vi "实时小时数据单参数上传2.vi"(11 "错误输入（无错误）":errorcluster) -> (4 "数据发送起始时间":timestamp format="%<%.3X\n%Y/%m/%d>T", 15 "error out":errorcluster)   [LabVIEW 2016, in "数据传输系统-04.lvlib"]
uses:
  <vilib>/Utility/config.llb/Read Key (String).vi
  <vilib>/Utility/config.llb/Write Key (String).vi
  <vilib>/Utility/config.llb/NI_LVConfig.lvlib
panel:
  out "数据拆分":bool
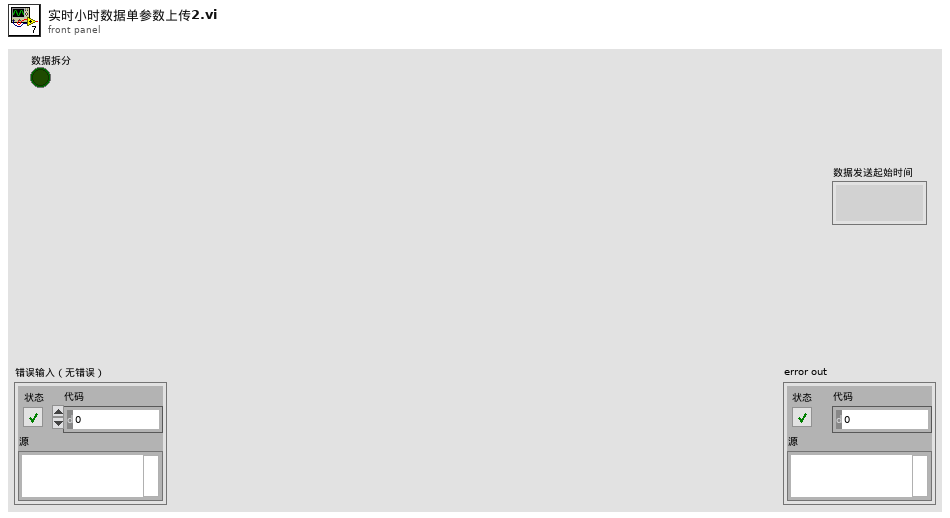
[diagram p1: front panel]
types:
  T1 = cluster{"CODMn":string, "CODCr":string, "DO":string, "铜":string, "PH":string, "氨氮":string, "比电导率":string, "水温":string, "COD":string, "浊度":string, "总氮":string, "总磷":string, "叶绿素a":string, "藻密度":string, "水位":string, "流速":string, "方向":string, "瞬时流量":string, "累积流量":string, "正累积流量":string, "负累积流量":string, "亚硝酸盐":string, "硫化物":string, "ORP":string, "铅":string, "镉":string, "锌":string, "镍":string, "锰":string, "汞":string, "气温":string, "气压":string, "风速":string, "风向":string, "空气温度":string, "相对湿度":string, "分钟雨量":string, "小时雨量":string, "日雨量":string, "累积雨量":string, "盐度":string, "磷酸盐":string, "硝氮":string, "氟化物":string, "挥发酚":string, "氯化物":string, "蓝绿藻":string, "余氯":string, "综合生物毒性":string, "艏向":string, "横摇":string, "纵摇":string, "分层标志":string, "层状态1":string, "层状态2":string, "水平平均流速":string, "流向":string, "北向流速分量":string, "东向流速分量":string, "垂直流速分量":string, "最大波高":string, "最大波周期":string, "1/10波高":string, "1/10波周期":string, "有效波高":string, "有效波周期":string, "平均波高":string, "平均波周期":string, "波向":string, "波个数":string, "水深":string, "X轴流速":string, "Y轴流速":string, "信号强度":string, "电压":string, "悬浮物":string}
  T2 = cluster{"setini":string, "sysini":string, "hechaini":string, "actualwrite":string, "actualread":string, "datasent":string, "反控命令信息队列":string, "反控与仪器交互":string}
  T3 = typedef "NI_LVConfig.lvlib/Config Data RefNum.ctl" = refnum<k1>
  T4 = cluster{"time1":string, "time2":string, "time3":string, "time4":string, "time5":string, "time6":string, "time7":string, "time8":string, "time9":string, "time10":string, "time11":string, "time12":string, "time13":string, "time14":string, "time15":string, "time16":string, "time17":string, "time18":string, "time19":string, "time20":string, "time21":string, "time22":string, "time23":string, "time24":string, "time25":string, "time26":string, "time27":string, "time28":string, "time29":string, "time30":string, "time31":string, "time32":string, "time33":string, "time34":string, "time35":string, "time36":string, "time37":string, "time38":string, "time39":string, "time40":string, "time41":string, "time42":string, "time43":string, "time44":string, "time45":string, "time46":string, "time47":string, "time48":string, "time49":string, "time50":string, "time51":string, "time52":string, "time53":string, "time54":string, "time55":string, "time56":string, "time57":string, "time58":string, "time59":string, "time60":string, "time61":string, "time62":string, "time63":string, "time64":string, "time65":string, "time66":string, "time67":string, "time68":string, "time69":string, "time70":string, "time71":string, "time72":string, "time73":string, "time74":string, "time75":string, "time76":string}
  T5 = cluster{"水样数据索引[0]":string, "水样数据索引[1]":string, "水样数据索引[2]":string, "水样数据索引[3]":string, "水样数据索引[4]":string, "水样数据索引[5]":string, "水样数据索引[6]":string, "水样数据索引[7]":string, "水样数据索引[8]":string, "水样数据索引[9]":string, "水样数据索引[10]":string, "水样数据索引[11]":string, "水样数据索引[12]":string, "水样数据索引[13]":string, "水样数据索引[14]":string, "水样数据索引[15]":string, "水样数据索引[16]":string, "水样数据索引[17]":string, "水样数据索引[18]":string, "水样数据索引[19]":string, "水样数据索引[20]":string, "水样数据索引[21]":string, "水样数据索引[22]":string, "水样数据索引[23]":string, "水样数据索引[24]":string, "水样数据索引[25]":string, "水样数据索引[26]":string, "水样数据索引[27]":string, "水样数据索引[28]":string, "水样数据索引[29]":string, "水样数据索引[30]":string, "水样数据索引[31]":string, "水样数据索引[32]":string, "水样数据索引[33]":string, "水样数据索引[34]":string, "水样数据索引[35]":string, "水样数据索引[36]":string, "水样数据索引[37]":string, "水样数据索引[38]":string, "水样数据索引[39]":string, "水样数据索引[40]":string, "水样数据索引[41]":string, "水样数据索引[42]":string, "水样数据索引[43]":string, "水样数据索引[44]":string, "水样数据索引[45]":string, "水样数据索引[46]":string, "水样数据索引[47]":string, "水样数据索引[48]":string, "水样数据索引[49]":string, "水样数据索引[50]":string, "水样数据索引[51]":string, "水样数据索引[52]":string, "水样数据索引[53]":string, "水样数据索引[54]":string, "水样数据索引[55]":string, "水样数据索引[56]":string, "水样数据索引[57]":string, "水样数据索引[58]":string, "水样数据索引[59]":string, "水样数据索引[60]":string, "水样数据索引[61]":string, "水样数据索引[62]":string, "水样数据索引[63]":string, "水样数据索引[64]":string, "水样数据索引[65]":string, "水样数据索引[66]":string, "水样数据索引[67]":string, "水样数据索引[68]":string, "水样数据索引[69]":string, "水样数据索引[70]":string, "水样数据索引[71]":string, "水样数据索引[72]":string, "水样数据索引[73]":string, "水样数据索引[74]":string, "水样数据索引[75]":string}
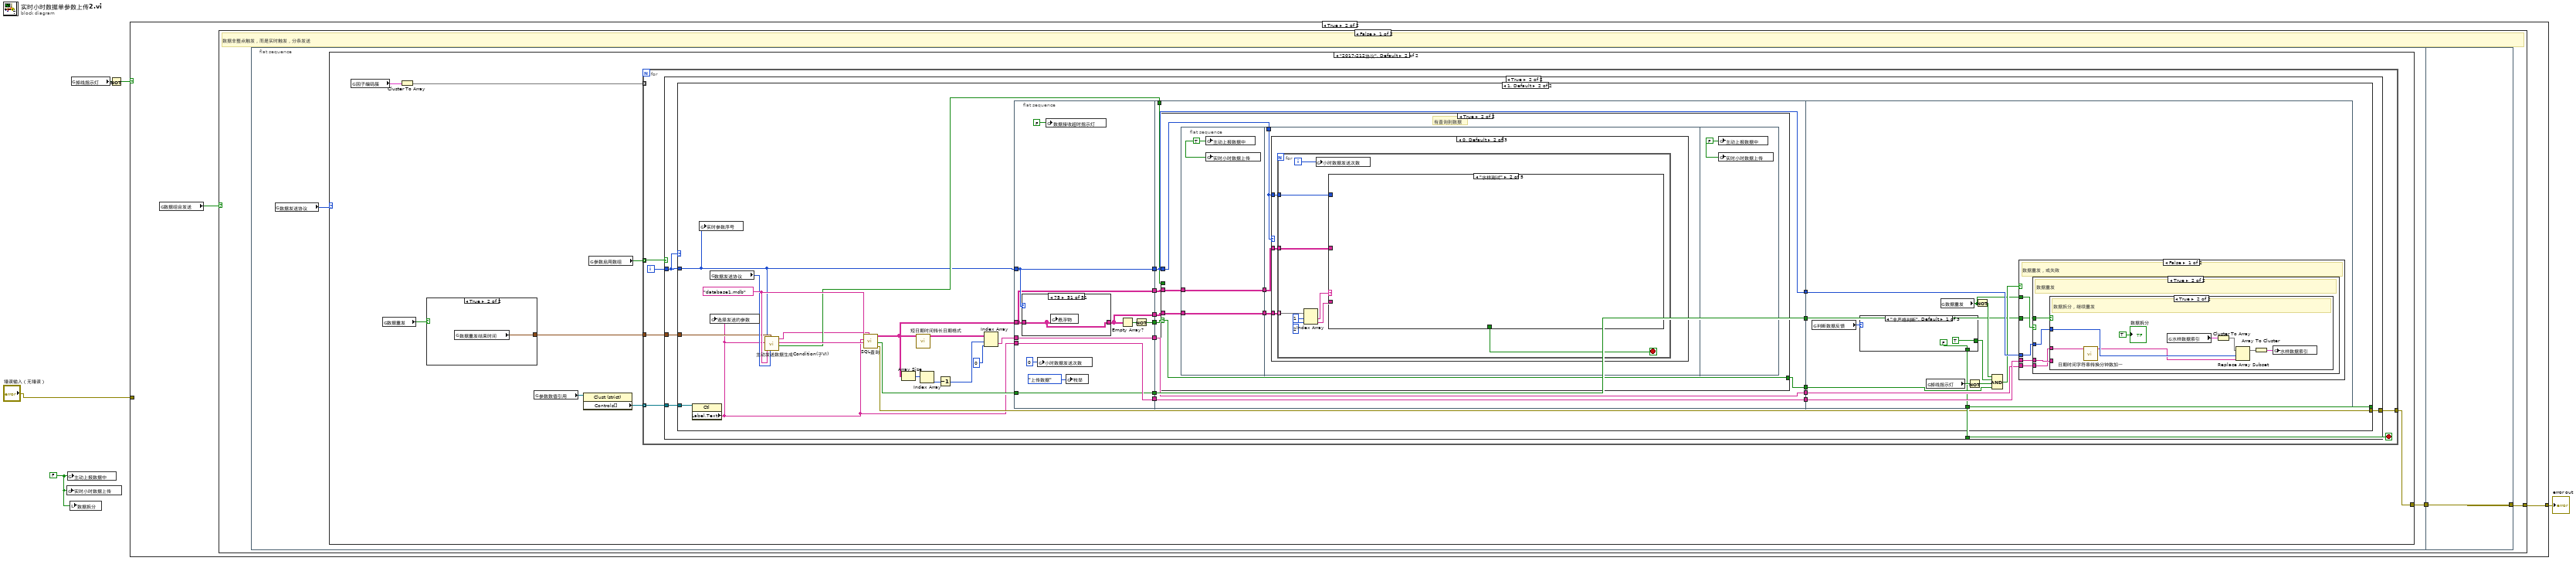
[diagram p0: block diagram]
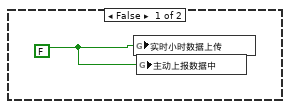
[diagram p2: hidden frame]
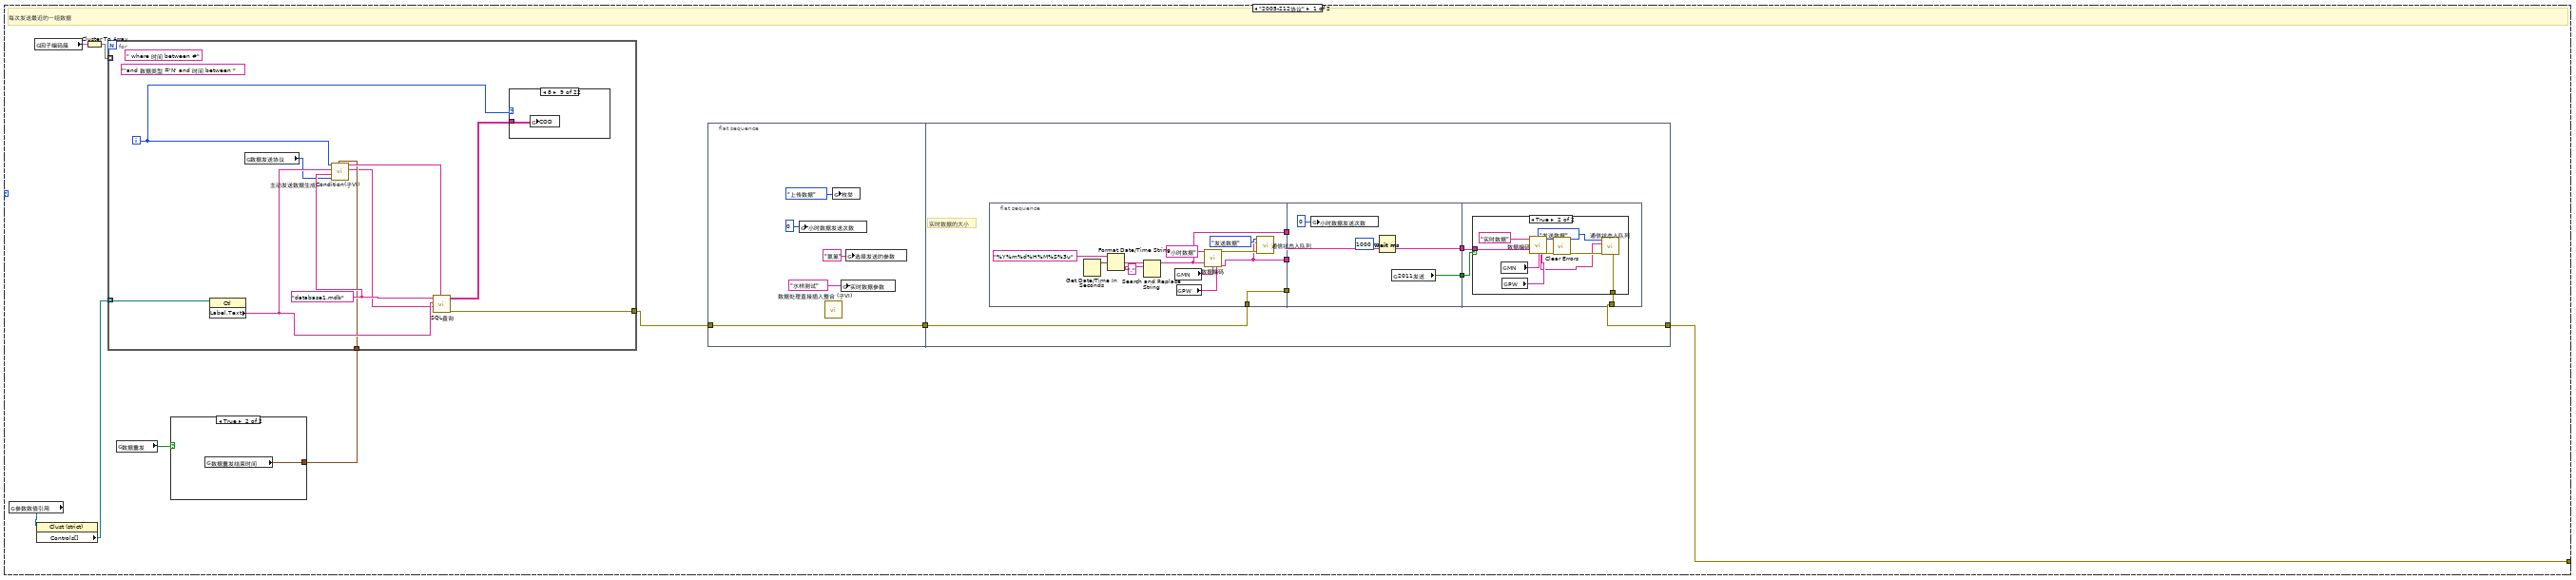
[diagram p3: hidden frame]
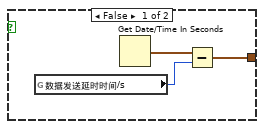
[diagram p4: hidden frame]
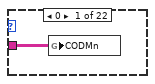
[diagram p6: hidden frame]
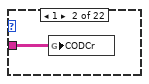
[diagram p7: hidden frame]
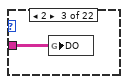
[diagram p8: hidden frame]
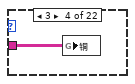
[diagram p9: hidden frame]
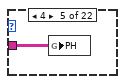
[diagram p10: hidden frame]
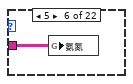
[diagram p11: hidden frame]
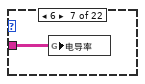
[diagram p12: hidden frame]
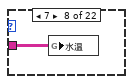
[diagram p13: hidden frame]
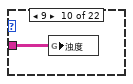
[diagram p14: hidden frame]
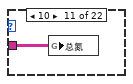
[diagram p15: hidden frame]
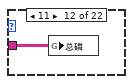
[diagram p16: hidden frame]
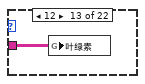
[diagram p17: hidden frame]
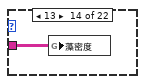
[diagram p18: hidden frame]
diagram:
  w1 = FALSE ("小时数据上传")
  n1 = global write "全局1.vi" "实时小时数据上传"(w1) -> ()
  n2 = global write "全局 数据发送重叠.vi" "主动上报数据中"(w1) -> ()
  n3 = local write "数据拆分"(w1) -> ()
  n4 = global read "全局 数据发送重叠.vi" "掉线指示灯"() -> (w5:bool)
  n5 = Not(x=w5) -> (.not. x?=w4:bool)
  n6 = case shown="True" w4 {
    tunnel: [_ w8] -> w3
    tunnel: "错误输入（无错误）" -> [_ _]
    frame False {
      w6 = FALSE ("小时数据上传")
      n7 = global write "全局1.vi" "实时小时数据上传"(w6) -> ()
      n8 = global write "全局 数据发送重叠.vi" "主动上报数据中"(w6) -> ()
    }
    frame True {
      n9 = global read "断电保存全局.vi" "数据组合发送"() -> (w7:bool)
      n10 = case shown="False" w7 {
        tunnel: [w9 _] -> w8
        frame False {
          # "数据非整点触发，而是实时触发，分条发送"
          n11 = flat-sequence {
            tunnel: [w12] -> w10
            tunnel: [w415] -> w9
            tunnel: w10 -> [w415]
            frame #0 {
              n12 = global read "断电保存全局.vi" "数据发送协议"() -> (w11:enum16{"2005-212协议", "2017-212协议"})
              n13 = case shown="\"2017-212协议\", Default" w11 {
                tunnel: [w17 w99] -> w12
                frame "2005-212协议" {
                  # "每次发送最近的一组数据"
                  n14 = global read "断电保存全局.vi" "参数数值引用"() -> (w15:refnum<vi>)
                  n15 = global read "断电保存全局.vi" "因子编码簇"() -> (w16:T1)
                  n16 = property class="Clust (strict)"(reference=w15) -> ("Controls[]"=w18:refnum<vi>[])  [unwired: 1 in, 2 out]
                  n17 = Cluster To Array(cluster=w16) -> (array=w21:string[])
                  n18 = global read "断电保存全局.vi" "数据重发"() -> (w14:bool)
                  n19 = case shown="True" w14 {
                    tunnel: [w22 w25] -> w13
                    frame False {
                      n20 = global read "断电保存全局.vi" "数据发送延时时间/s"() -> (w23:i32)
                      n21 = Get Date/Time In Seconds() -> (seconds since 1Jan1904=w24:timestamp)
                      n22 = Subtract(x=w24, y=w23) -> (x-y=w22:timestamp)
                    }
                    frame True {
                      n23 = global read "断电保存全局.vi" "数据重发结束时间"() -> (w25:timestamp)
                    }
                  }
                  n24 = for {
                    tunnel: w21 -> [_] mode=indexing
                    tunnel: [w75] -> w20
                    tunnel: w18 -> [w70] mode=indexing
                    tunnel: w13 -> [w67]
                    i -> [w68]
                    (unwired) " where 时间 between #"
                    w73 = "database1.mdb" ("database")
                    (unwired) "'and 数据类型 ='N' and 时间 between "
                    n25 = property class="Ctl"(reference=w70) -> ("Label.Text"=w74:string)  [unwired: 1 in, 2 out]
                    n26 = global read "断电保存全局.vi" "数据发送协议"() -> (w71:enum16{"2005-212协议", "2017-212协议"})
                    n27 = call "主动发送数据生成Condition(子VI).vi"("结束时间"=w67, "数据发送协议"=w71, "database"=w73, "Label.Text"=w74, "数值"=w68) -> ("columns"=w66:string[], "CONDITION"=w72:string)  [unwired: 3 in, 2 out]
                    n28 = call "SQL查询.vi"("condition"=w72, "columns"=w66, "table输入"=w74, "database"=w73) -> ("error out"=w75:errorcluster, "data"=w69:string[][])  [unwired: 4 in, 2 out]
                    n29 = case shown="8" w68 {
                      tunnel: w69 -> [w76 w77 w78 w79 w80 w81 w82 w83 w84 w85 w86 w87 w88 w89 _ _ _ _ w90 w91 w92 _]
                      frame 0 {
                        n30 = global write "全局 所有参数.vi" "CODMn"(w76) -> ()
                      }
                      frame 1 {
                        n31 = global write "全局 所有参数.vi" "CODCr"(w77) -> ()
                      }
                      frame 2 {
                        n32 = global write "全局 所有参数.vi" "DO"(w78) -> ()
                      }
                      frame 3 {
                        n33 = global write "全局 所有参数.vi" "铜"(w79) -> ()
                      }
                      frame 4 {
                        n34 = global write "全局 所有参数.vi" "PH"(w80) -> ()
                      }
                      frame 5 {
                        n35 = global write "全局 所有参数.vi" "氨氮"(w81) -> ()
                      }
                      frame 6 {
                        n36 = global write "全局 所有参数.vi" "电导率"(w82) -> ()
                      }
                      frame 7 {
                        n37 = global write "全局 所有参数.vi" "水温"(w83) -> ()
                      }
                      frame 8 {
                        n38 = global write "全局 所有参数.vi" "COD"(w84) -> ()
                      }
                      frame 9 {
                        n39 = global write "全局 所有参数.vi" "浊度"(w85) -> ()
                      }
                      frame 10 {
                        n40 = global write "全局 所有参数.vi" "总氮"(w86) -> ()
                      }
                      frame 11 {
                        n41 = global write "全局 所有参数.vi" "总磷"(w87) -> ()
                      }
                      frame 12 {
                        n42 = global write "全局 所有参数.vi" "叶绿素"(w88) -> ()
                      }
                      frame 13 {
                        n43 = global write "全局 所有参数.vi" "藻密度"(w89) -> ()
                      }
                      frame 14 {
                      }
                      frame 15 {
                      }
                      frame 16 {
                      }
                      frame 17 {
                      }
                      frame 18 {
                        n44 = global write "全局 所有参数.vi" "亚硝酸盐"(w90) -> ()
                      }
                      frame 19 {
                        n45 = global write "全局 所有参数.vi" "硫化物"(w91) -> ()
                      }
                      frame 20 {
                        n46 = global write "全局 所有参数.vi" "ORP"(w92) -> ()
                      }
                      frame 21, Default {
                      }
                    }
                  }
                  n47 = flat-sequence {
                    tunnel: w20 -> [w26]
                    tunnel: [w26] -> w19
                    tunnel: w19 -> [w35]
                    tunnel: [w34] -> w17
                    frame #0 {
                      n48 = global write "全局 小时数据发送次数.vi" "小时数据发送次数"(0 ("小时数据发送次数")) -> ()
                      n49 = call "数据处理直接插入整合 (子VI).vi"() -> ()  [unwired: 12 in]
                      n50 = global write "全局1.vi" "枚举"(enum16{"返回请求应答", "上传数据", "返回执行结果"}."上传数据" ("枚举")) -> ()
                      n51 = global write "全局 实时数据参数.vi" "实时数据参数"("水样测试" ("实时数据参数")) -> ()
                      n52 = global write "全局 水样时间.vi" "选择发送的参数"("氨氮" ("选择发送的参数")) -> ()
                    }
                    frame #1 {
                      # "实时数据的大小"
                      n53 = flat-sequence {
                        tunnel: [w38] -> w37
                        tunnel: [w41] -> w36
                        tunnel: w35 -> [w41]
                        tunnel: [w40] -> w33
                        tunnel: w37 -> [_]
                        tunnel: w36 -> [_]
                        tunnel: w33 -> [w51]
                        tunnel: [w51] -> w32
                        tunnel: [w50] -> w31
                        tunnel: [w56] -> w34
                        tunnel: w32 -> [w55]
                        tunnel: w31 -> [w54]
                        frame #0 {
                          n54 = Get Date/Time In Seconds() -> (seconds since 1Jan1904=w47:timestamp)
                          n55 = Format Date/Time String(time format string (%c)="%Y%m%d%H%M%S%3u" ("时间格式字符串(%c)"), seconds (now)=w47) -> (date/time string=w48:string)  [unwired: 1 in]
                          n56 = Search and Replace String(input string=w48, search string="." ("搜索字符串")) -> (result string=w40:string)  [unwired: 6 in, 3 out]
                          n57 = global read "断电保存全局.vi" "MN"() -> (w44:string)
                          n58 = global read "断电保存全局.vi" "PW"() -> (w43:string)
                          n59 = call "数据编码.vi"("table输入"="小时数据" ("新元素/子数组"), "QN"=w40, "MN"=w44, "PW"=w43) -> ("错误常量"=w42:errorcluster, "通讯包字符串"=w38:string)  [unwired: 10 in]
                          n60 = call "通信状态入队列.vi"("错误输入（无错误）"=w42, "发送报文"=w38, "枚举"=enum16{"打开连接", "发送数据", "读取数据", "数据处理", "关闭连接"}."发送数据") -> ()  [unwired: 8 in, 1 out]
                        }
                        frame #1 {
                          n61 = global write "全局 小时数据发送次数.vi" "小时数据发送次数"(0 ("小时数据发送次数")) -> ()
                          n62 = Wait (ms)(milliseconds to wait=u32 1000 ("等待时间（毫秒）")) -> ()  [unwired: 1 out]
                          n63 = global read "断电保存全局.vi" "2011发送"() -> (w50:bool)
                        }
                        frame #2 {
                          n64 = case shown="True" w54 {
                            tunnel: [_ w61] -> w56
                            tunnel: w55 -> [_ w60]
                            frame False {
                            }
                            frame True {
                              n65 = global read "断电保存全局.vi" "MN"() -> (w63:string)
                              n66 = global read "断电保存全局.vi" "PW"() -> (w64:string)
                              n67 = call "数据编码.vi"("table输入"="实时数据" ("新元素/子数组"), "QN"=w60, "MN"=w63, "PW"=w64) -> ("错误常量"=w62:errorcluster, "通讯包字符串"=w57:string)  [unwired: 10 in]
                              n68 = call <vilib>:"Clear Errors.vi"("error in (no error)"=w62) -> ("error out"=w59:errorcluster)  [unwired: 5 in, 1 out]
                              n69 = call "通信状态入队列.vi"("错误输入（无错误）"=w59, "发送报文"=w57, "枚举"=enum16{"打开连接", "发送数据", "读取数据", "数据处理", "关闭连接"}."发送数据") -> ("错误输出"=w61:errorcluster)  [unwired: 8 in]
                            }
                          }
                        }
                      }
                    }
                  }
                }
                frame "2017-212协议", Default {
                  n70 = global read "断电保存全局.vi" "因子编码簇"() -> (w97:T1)
                  n71 = global read "断电保存全局.vi" "数据重发"() -> (w94:bool)
                  n72 = Cluster To Array(cluster=w97) -> (array=w100:string[])
                  n73 = case shown="True" w94 {
                    tunnel: [w102 w105] -> w93
                    frame False {
                      n74 = global read "断电保存全局.vi" "数据发送延时时间/s"() -> (w103:i32)
                      n75 = global write "断电保存全局.vi" "2011发送"(TRUE ("2011发送")) -> ()
                      n76 = Get Date/Time In Seconds() -> (seconds since 1Jan1904=w104:timestamp)
                      n77 = Subtract(x=w104, y=w103) -> (x-y=w102:timestamp)
                    }
                    frame True {
                      n78 = global read "断电保存全局.vi" "数据重发结束时间"() -> (w105:timestamp)
                    }
                  }
                  n79 = global read "断电保存全局.vi" "参数数值引用"() -> (w96:refnum<vi>)
                  n80 = property class="Clust (strict)"(reference=w96) -> ("Controls[]"=w98:refnum<vi>[])  [unwired: 1 in, 2 out]
                  n81 = global read "断电保存全局.vi" "参数启用数组"() -> (w95:bool[])
                  n82 = for {
                    tunnel: w100 -> [_] mode=indexing
                    tunnel: [w111] -> w99
                    tunnel: w98 -> [w110] mode=indexing
                    tunnel: w95 -> [w109] mode=indexing
                    tunnel: w93 -> [w108]
                    i -> [w106]
                    stop <- w107 stop-if-true
                    n83 = case shown="True" w109 {
                      tunnel: [_ w116] -> w111
                      tunnel: w106 -> [_ w112]
                      tunnel: w110 -> [_ w115]
                      tunnel: w108 -> [_ w114]
                      tunnel: [_ w113] -> w107
                      frame False {
                      }
                      frame True {
                        n84 = case shown="1, Default" w112 {
                          tunnel: [_ w135] -> w116
                          tunnel: w115 -> [_ w128]
                          tunnel: w114 -> [_ w126]
                          tunnel: [FALSE ("数据接收超时指示灯") w125] -> w113
                          tunnel: w112 -> [_ w118]
                          frame 16..20 {
                          }
                          frame 1, Default {
                            w134 = "database1.mdb" ("database")
                            n85 = property class="Ctl"(reference=w128) -> ("Label.Text"=w121:string)  [unwired: 1 in, 2 out]
                            n86 = global write "断电保存全局.vi" "实时参数序号"(w118) -> ()
                            n87 = global read "断电保存全局.vi" "数据发送协议"() -> (w133:enum16{"2005-212协议", "2017-212协议"})
                            n88 = global write "全局 水样时间.vi" "选择发送的参数"(w121) -> ()
                            n89 = call "主动发送数据生成Condition(子VI).vi"("结束时间"=w126, "数据发送协议"=w133, "database"=w134, "Label.Text"=w121, "数值"=w118) -> ("database溢出"=w122:bool, "columns"=w127:string[], "CONDITION"=w119:string)  [unwired: 3 in, 1 out]
                            n90 = call "SQL查询.vi"("condition"=w119, "columns"=w127, "table输入"=w121, "database"=w134) -> ("error out"=w135:errorcluster, "拆分数据"=w124:bool, "data"=w120:string[][])  [unwired: 4 in, 1 out]
                            n91 = Array Size(array=w120) -> (size(s)=w132:i32[])
                            n92 = call "短日期时间转长日期格式.vi"("data"=w120) -> ("输出数组"=w136:string[][])  [unwired: 10 in]
                            n93 = Index Array(array=w132) -> (element=w131:i32)  [unwired: 1 in]
                            n94 = Decrement(x=w131) -> (x-1=w130:i32)
                            n95 = Index Array(array=w136, index (row)=w130, index (col)=0 ("禁用的索引 (列)")) -> (element=w123:string)
                            n96 = flat-sequence {
                              tunnel: [w152] -> w148
                              tunnel: [w149] -> w147
                              tunnel: w120 -> [w151]
                              tunnel: w118 -> [w155]
                              tunnel: w121 -> [w157]
                              tunnel: [w157] -> w146
                              tunnel: w123 -> [w156]
                              tunnel: [w156] -> w145
                              tunnel: [w155] -> w144
                              tunnel: [w151] -> w143
                              tunnel: [w150] -> w142
                              tunnel: w124 -> [w150]
                              tunnel: w148 -> [w216]
                              tunnel: w147 -> [w219]
                              tunnel: [w218] -> w141
                              tunnel: w146 -> [w218]
                              tunnel: [w211] -> w140
                              tunnel: w145 -> [w211]
                              tunnel: [w217] -> w139
                              tunnel: w144 -> [w217]
                              tunnel: [w213] -> w138
                              tunnel: w143 -> [w215]
                              tunnel: w142 -> [w214]
                              tunnel: [w214] -> w137
                              tunnel: w122 -> [w212]
                              tunnel: w141 -> [w356]
                              tunnel: w140 -> [w355]
                              tunnel: w139 -> [w354]
                              tunnel: w138 -> [w353]
                              tunnel: [w345] -> w125
                              tunnel: w137 -> [w344]
                              frame #0 {
                                n97 = case shown="75" w155 {
                                tunnel: w151 -> [w160 w161 w162 w163 w164 w165 w166 w167 w168 w169 w170 w171 w172 w173 w174 _ _ _ _ _ _ _ w182 w183 w184 w185 w186 w187 w188 w189 w190 _ _ _ _ _ _ _ _ _ _ w201 w202 w203 w204 w205 w206 w207 w208 w209 w210]
                                tunnel: [w160 w161 w162 w163 w164 w165 w166 w167 w168 w169 w170 w171 w172 w173 w174 w175 w176 w177 w178 w179 w180 w181 w182 w183 w184 w185 w186 w187 w188 w189 w190 w191 w192 w193 w194 w195 w196 w197 w198 w199 w200 w201 w202 w203 w204 w205 w206 w207 w208 w209 w210] -> w149
                                frame 999, Default {
                                }
                                frame 0 {
                                n98 = global write "全局 所有参数.vi" "CODMn"(w161) -> ()
                                }
                                frame 1 {
                                n99 = global write "全局 所有参数.vi" "CODCr"(w162) -> ()
                                }
                                frame 2 {
                                n100 = global write "全局 所有参数.vi" "DO"(w163) -> ()
                                }
                                frame 3 {
                                n101 = global write "全局 所有参数.vi" "铜"(w164) -> ()
                                }
                                frame 4 {
                                n102 = global write "全局 所有参数.vi" "PH"(w165) -> ()
                                }
                                frame 5 {
                                n103 = global write "全局 所有参数.vi" "氨氮"(w166) -> ()
                                }
                                frame 6 {
                                n104 = global write "全局 所有参数.vi" "电导率"(w167) -> ()
                                }
                                frame 7 {
                                n105 = global write "全局 所有参数.vi" "水温"(w168) -> ()
                                }
                                frame 8 {
                                n106 = global write "全局 所有参数.vi" "COD"(w169) -> ()
                                }
                                frame 9 {
                                n107 = global write "全局 所有参数.vi" "浊度"(w170) -> ()
                                }
                                frame 10 {
                                n108 = global write "全局 所有参数.vi" "总氮"(w171) -> ()
                                }
                                frame 11 {
                                n109 = global write "全局 所有参数.vi" "总磷"(w172) -> ()
                                }
                                frame 12 {
                                n110 = global write "全局 所有参数.vi" "叶绿素"(w173) -> ()
                                }
                                frame 13 {
                                n111 = global write "全局 所有参数.vi" "藻密度"(w174) -> ()
                                }
                                frame 14 {
                                n112 = global read "全局 所有参数.vi" "水位"() -> (w175:string[][])
                                }
                                frame 15 {
                                n113 = global read "全局 所有参数.vi" "流速"() -> (w176:string[][])
                                }
                                frame 16 {
                                n114 = global read "全局 所有参数.vi" "方向"() -> (w177:string[][])
                                }
                                frame 17 {
                                n115 = global read "全局 所有参数.vi" "瞬时流量"() -> (w178:string[][])
                                }
                                frame 18 {
                                n116 = global read "全局 所有参数.vi" "累积流量"() -> (w179:string[][])
                                }
                                frame 19 {
                                n117 = global read "全局 所有参数.vi" "正累积流量"() -> (w180:string[][])
                                }
                                frame 20 {
                                n118 = global read "全局 所有参数.vi" "负累积流量"() -> (w181:string[][])
                                }
                                frame 21 {
                                n119 = global write "全局 所有参数.vi" "亚硝酸盐"(w182) -> ()
                                }
                                frame 22 {
                                n120 = global write "全局 所有参数.vi" "硫化物"(w183) -> ()
                                }
                                frame 23 {
                                n121 = global write "全局 所有参数.vi" "ORP"(w184) -> ()
                                }
                                frame 24 {
                                n122 = global write "全局 所有参数.vi" "铅"(w185) -> ()
                                }
                                frame 25 {
                                n123 = global write "全局 所有参数.vi" "镉"(w186) -> ()
                                }
                                frame 26 {
                                n124 = global write "全局 所有参数.vi" "锌"(w187) -> ()
                                }
                                frame 27 {
                                n125 = global write "全局 所有参数.vi" "镍"(w188) -> ()
                                }
                                frame 28 {
                                n126 = global write "全局 所有参数.vi" "锰"(w189) -> ()
                                }
                                frame 29 {
                                n127 = global write "全局 所有参数.vi" "汞"(w190) -> ()
                                }
                                frame 30 {
                                n128 = global read "全局 所有参数.vi" "气温"() -> (w191:string[][])
                                }
                                frame 31 {
                                n129 = global read "全局 所有参数.vi" "气压"() -> (w192:string[][])
                                }
                                frame 32 {
                                n130 = global read "全局 所有参数.vi" "风速"() -> (w193:string[][])
                                }
                                frame 33 {
                                n131 = global read "全局 所有参数.vi" "风向"() -> (w194:string[][])
                                }
                                frame 34 {
                                n132 = global read "全局 所有参数.vi" "空气温度"() -> (w195:string[][])
                                }
                                frame 35 {
                                n133 = global read "全局 所有参数.vi" "相对湿度"() -> (w196:string[][])
                                }
                                frame 36 {
                                n134 = global read "全局 所有参数.vi" "分钟雨量"() -> (w197:string[][])
                                }
                                frame 37 {
                                n135 = global read "全局 所有参数.vi" "小时雨量"() -> (w198:string[][])
                                }
                                frame 38 {
                                n136 = global read "全局 所有参数.vi" "日雨量"() -> (w199:string[][])
                                }
                                frame 39 {
                                n137 = global read "全局 所有参数.vi" "累积雨量"() -> (w200:string[][])
                                }
                                frame 40 {
                                n138 = global write "全局 所有参数.vi" "盐度"(w201) -> ()
                                }
                                frame 41 {
                                n139 = global write "全局 所有参数.vi" "磷酸盐"(w202) -> ()
                                }
                                frame 42 {
                                n140 = global write "全局 所有参数.vi" "硝氮"(w203) -> ()
                                }
                                frame 43 {
                                n141 = global write "全局 所有参数.vi" "氟化物"(w204) -> ()
                                }
                                frame 44 {
                                n142 = global write "全局 所有参数.vi" "挥发酚"(w205) -> ()
                                }
                                frame 45 {
                                n143 = global write "全局 所有参数.vi" "氯化物"(w206) -> ()
                                }
                                frame 46 {
                                n144 = global write "全局 所有参数.vi" "蓝绿藻"(w207) -> ()
                                }
                                frame 47 {
                                n145 = global write "全局 所有参数.vi" "余氯"(w208) -> ()
                                }
                                frame 48 {
                                n146 = global write "全局 所有参数.vi" "综合生物毒性"(w209) -> ()
                                }
                                frame 75 {
                                n147 = global write "全局 所有参数.vi" "悬浮物"(w210) -> ()
                                }
                                }
                                n148 = global write "全局 小时数据发送次数.vi" "小时数据发送次数"(0 ("小时数据发送次数")) -> ()
                                n149 = global write "全局 数据发送重叠.vi" "数据接收超时指示灯"(FALSE ("数据接收超时指示灯")) -> ()
                                n150 = global write "全局1.vi" "枚举"(enum16{"返回请求应答", "上传数据", "返回执行结果"}."上传数据" ("枚举")) -> ()
                                n151 = Empty Array?(array=w149) -> (empty?=w153:bool)
                                n152 = Not(x=w153) -> (.not. x?=w152:bool)
                              }
                              frame #1 {
                                n153 = case shown="True" w216 {
                                selector: w216 -> [_ w221]
                                tunnel: w219 -> [_ w226]
                                tunnel: w217 -> [_ w225]
                                tunnel: w215 -> [_ w223]
                                tunnel: [w220 w221] -> w213
                                tunnel: w212 -> [w220 _]
                                frame False {
                                }
                                frame True {
                                # "有查询到数据"
                                n154 = flat-sequence {
                                tunnel: w226 -> [w229]
                                tunnel: [w229] -> w224
                                tunnel: w223 -> [w227]
                                tunnel: [w227] -> w222
                                tunnel: w225 -> [w231]
                                tunnel: w224 -> [w232]
                                tunnel: w222 -> [w230]
                                frame #0 {
                                w228 = TRUE ("小时数据上传")
                                n155 = global write "全局 数据发送重叠.vi" "主动上报数据中"(w228) -> ()
                                n156 = global write "全局1.vi" "实时小时数据上传"(w228) -> ()
                                }
                                frame #1 {
                                n157 = case shown="0, Default" w231 {
                                selector: w231 -> [w234 _ _]
                                tunnel: w231 -> [_ w278 w339]
                                tunnel: w232 -> [w236 w277 w338]
                                tunnel: w230 -> [w233 w276 w337]
                                frame 16..20, 30..39 {
                                n158 = for {
                                tunnel: [w271] -> w237
                                tunnel: w234 -> [w269]
                                tunnel: w236 -> [_] mode=indexing
                                i -> [w272]
                                stop <- w270 stop-if-true
                                n159 = case shown="16..20" w269 {
                                tunnel: [w275 _] -> w271
                                tunnel: w269 -> [w274 _]
                                tunnel: [w273 _] -> w270
                                frame 0, Default {
                                n160 = call "小时数据发送 (子VI).vi"("数值"=w274) -> ("error out"=w275:errorcluster, "超时退出"=w273:bool)  [unwired: 9 in]
                                }
                                frame 16..20 {
                                }
                                }
                                n161 = global write "全局 小时数据发送次数.vi" "小时数据发送次数"(w272) -> ()
                                }
                                n162 = global read "断电保存全局.vi" "2011发送"() -> (w235:bool)
                                n163 = case shown="True" w235 {
                                tunnel: w237 -> [_ w242]
                                tunnel: w234 -> [_ w241]
                                tunnel: w233 -> [_ w240]
                                tunnel: w234 -> [_ w238]
                                frame False {
                                }
                                frame True {
                                n164 = flat-sequence {
                                tunnel: w242 -> [w246]
                                tunnel: [w246] -> w243
                                tunnel: w241 -> [w245]
                                tunnel: w240 -> [w244]
                                tunnel: [w244] -> w239
                                frame #0 {
                                n165 = case shown="30" w245 {
                                tunnel: w244 -> [_ w247 w248 w249 w250 w251 w252 w253 w254 w255 w256 w257 w258 w259 w260 w261 w262 w263]
                                frame 0, Default {
                                }
                                frame 14 {
                                n166 = global write "全局 所有参数.vi" "水位"(w247) -> ()
                                }
                                frame 15 {
                                n167 = global write "全局 所有参数.vi" "流速"(w248) -> ()
                                }
                                frame 16 {
                                n168 = global write "全局 所有参数.vi" "方向"(w249) -> ()
                                }
                                frame 17 {
                                n169 = global write "全局 所有参数.vi" "瞬时流量"(w250) -> ()
                                }
                                frame 18 {
                                n170 = global write "全局 所有参数.vi" "累积流量"(w251) -> ()
                                }
                                frame 19 {
                                n171 = global write "全局 所有参数.vi" "正累积流量"(w252) -> ()
                                }
                                frame 20 {
                                n172 = global write "全局 所有参数.vi" "负累积流量"(w253) -> ()
                                }
                                frame 30 {
                                n173 = global write "全局 所有参数.vi" "气温"(w254) -> ()
                                }
                                frame 31 {
                                n174 = global write "全局 所有参数.vi" "气压"(w255) -> ()
                                }
                                frame 32 {
                                n175 = global write "全局 所有参数.vi" "风速"(w256) -> ()
                                }
                                frame 33 {
                                n176 = global write "全局 所有参数.vi" "风向"(w257) -> ()
                                }
                                frame 34 {
                                n177 = global write "全局 所有参数.vi" "空气温度"(w258) -> ()
                                }
                                frame 35 {
                                n178 = global write "全局 所有参数.vi" "相对湿度"(w259) -> ()
                                }
                                frame 36 {
                                n179 = global write "全局 所有参数.vi" "分钟雨量"(w260) -> ()
                                }
                                frame 37 {
                                n180 = global write "全局 所有参数.vi" "小时雨量"(w261) -> ()
                                }
                                frame 38 {
                                n181 = global write "全局 所有参数.vi" "日雨量"(w262) -> ()
                                }
                                frame 39 {
                                n182 = global write "全局 所有参数.vi" "累积雨量"(w263) -> ()
                                }
                                }
                                }
                                }
                                n183 = for {
                                tunnel: w243 -> [_]
                                tunnel: w239 -> [_] mode=indexing
                                tunnel: w238 -> [w264]
                                i -> [w266]
                                stop <- w265 stop-if-true
                                n184 = case shown="14..20" w264 {
                                tunnel: w264 -> [w268 _]
                                tunnel: [w267 _] -> w265
                                frame 0, Default {
                                n185 = call "实时数据发送 (子VI).vi"("数值"=w268) -> ("超时退出"=w267:bool)  [unwired: 10 in]
                                }
                                frame 14..20 {
                                }
                                }
                                n186 = global write "全局 小时数据发送次数.vi" "小时数据发送次数"(w266) -> ()
                                }
                                }
                                }
                                }
                                frame 0, Default {
                                n187 = for {
                                tunnel: w278 -> [w281]
                                tunnel: w277 -> [w287] mode=indexing
                                tunnel: w276 -> [w283]
                                i -> [w282]
                                stop <- w279 stop-if-true
                                n188 = Index Array(array=w287, index #1=1 ("索引"), index #2=2 ("索引")) -> (element #1=w280:string, element #2=w284:string)
                                n189 = global write "全局 小时数据发送次数.vi" "小时数据发送次数"(w282) -> ()
                                n190 = case shown="\"水样测试\"" w280 {
                                tunnel: w281 -> [_ w291 _ _ _]
                                tunnel: w284 -> [_ w290 w329 w332 w335]
                                tunnel: w283 -> [_ w289 _ _ _]
                                tunnel: [_ w288 w328 w331 w334] -> w279
                                frame "假", Default {
                                }
                                frame "水样测试" {
                                n191 = case shown="\"hd\", \"N\", Default" w290 {
                                tunnel: w291 -> [w295 w319]
                                tunnel: w289 -> [w294 _]
                                tunnel: [w292 w321] -> w288
                                frame "M" {
                                n192 = global read "断电保存全局.vi" "2011发送"() -> (w293:bool)
                                n193 = case shown="True" w293 {
                                tunnel: w295 -> [_ w298]
                                tunnel: w294 -> [_ w297]
                                tunnel: [_ w296] -> w292
                                frame False {
                                }
                                frame True {
                                n194 = flat-sequence {
                                tunnel: w298 -> [w300]
                                tunnel: w297 -> [w301]
                                tunnel: [w300] -> w299
                                tunnel: w299 -> [w317]
                                tunnel: [w316] -> w296
                                frame #0 {
                                n195 = case shown="15" w300 {
                                tunnel: w301 -> [_ w302 w303 w304 w305 w306 w307 w308 w309 w310 w311 w312 w313 w314 w315]
                                frame 0, Default {
                                }
                                frame 14 {
                                n196 = global write "全局 所有参数.vi" "水位"(w302) -> ()
                                }
                                frame 15 {
                                n197 = global write "全局 所有参数.vi" "流速"(w303) -> ()
                                }
                                frame 16 {
                                n198 = global write "全局 所有参数.vi" "瞬时流量"(w304) -> ()
                                }
                                frame 17 {
                                n199 = global write "全局 所有参数.vi" "累积流量"(w305) -> ()
                                }
                                frame 27 {
                                n200 = global write "全局 所有参数.vi" "气温"(w306) -> ()
                                }
                                frame 28 {
                                n201 = global write "全局 所有参数.vi" "气压"(w307) -> ()
                                }
                                frame 29 {
                                n202 = global write "全局 所有参数.vi" "风速"(w308) -> ()
                                }
                                frame 30 {
                                n203 = global write "全局 所有参数.vi" "风向"(w309) -> ()
                                }
                                frame 31 {
                                n204 = global write "全局 所有参数.vi" "空气温度"(w310) -> ()
                                }
                                frame 32 {
                                n205 = global write "全局 所有参数.vi" "相对湿度"(w311) -> ()
                                }
                                frame 33 {
                                n206 = global write "全局 所有参数.vi" "分钟雨量"(w312) -> ()
                                }
                                frame 34 {
                                n207 = global write "全局 所有参数.vi" "小时雨量"(w313) -> ()
                                }
                                frame 35 {
                                n208 = global write "全局 所有参数.vi" "日雨量"(w314) -> ()
                                }
                                frame 36 {
                                n209 = global write "全局 所有参数.vi" "累积雨量"(w315) -> ()
                                }
                                }
                                }
                                frame #1 {
                                n210 = call "实时数据发送 (子VI).vi"("数值"=w317) -> ("超时退出"=w316:bool)  [unwired: 10 in]
                                }
                                }
                                }
                                }
                                }
                                frame "hd", "N", Default {
                                n211 = call "小时数据发送 (子VI).vi"("数值"=w319) -> ("error out"=w322:errorcluster, "超时退出"=w320:bool)  [unwired: 9 in]
                                n212 = global read "断电保存全局.vi" "2011发送"() -> (w318:bool)
                                n213 = case shown="False" w318 {
                                tunnel: w319 -> [_ w327]
                                tunnel: w322 -> [_ _]
                                tunnel: [w323 w324] -> w321
                                tunnel: w320 -> [w323 w326]
                                frame False {
                                }
                                frame True {
                                n214 = call "实时数据发送 (子VI).vi"("数值"=w327) -> ("超时退出"=w325:bool)  [unwired: 10 in]
                                n215 = Or(x=w326, y=w325) -> (x .or. y?=w324:bool)
                                }
                                }
                                }
                                }
                                }
                                frame "空白测试", "零点核查" {
                                n216 = case shown="\"N\", Default" w329 {
                                tunnel: [_ w330] -> w328
                                frame "M" {
                                }
                                frame "N", Default {
                                n217 = call "零点核查数据发送 (子VI).vi"() -> ("超时退出"=w330:bool)  [unwired: 11 in]
                                }
                                }
                                }
                                frame "跨度核查" {
                                n218 = case shown="\"N\", Default" w332 {
                                tunnel: [_ w333] -> w331
                                frame "M" {
                                }
                                frame "N", Default {
                                n219 = call "跨度核查数据发送 (子VI).vi"() -> ("超时退出"=w333:bool)  [unwired: 11 in]
                                }
                                }
                                }
                                frame "标样核查" {
                                n220 = case shown="\"N\", Default" w335 {
                                tunnel: [_ w336] -> w334
                                frame "M" {
                                }
                                frame "N", Default {
                                n221 = call "标样核查数据发送(子VI).vi"() -> ("超时退出"=w336:bool)  [unwired: 11 in]
                                }
                                }
                                }
                                }
                                }
                                }
                                frame 14, 15 {
                                n222 = for {
                                tunnel: w339 -> [w341]
                                tunnel: w338 -> [_] mode=indexing
                                tunnel: w337 -> [_]
                                i -> [w342]
                                stop <- w340 stop-if-true
                                n223 = global write "全局 小时数据发送次数.vi" "小时数据发送次数"(w342) -> ()
                                n224 = call "小时数据发送 (子VI).vi"("数值"=w341) -> ("超时退出"=w340:bool)  [unwired: 9 in, 1 out]
                                }
                                }
                                }
                                }
                                frame #2 {
                                w343 = FALSE ("小时数据上传")
                                n225 = global write "全局 数据发送重叠.vi" "主动上报数据中"(w343) -> ()
                                n226 = global write "全局1.vi" "实时小时数据上传"(w343) -> ()
                                }
                                }
                                }
                                }
                              }
                              frame #2 {
                                n227 = global read "断电保存全局.vi" "判断数据反馈"() -> (w350:enum16{"非严格判断", "严格判断", "不判断"})
                                n228 = case shown="\"非严格判断\", Default" w350 {
                                tunnel: [TRUE w360 TRUE] -> w349
                                tunnel: [FALSE ("数据接收超时指示灯") w359 FALSE ("数据接收超时指示灯")] -> w345
                                frame "非严格判断", Default {
                                }
                                frame "严格判断" {
                                n229 = global read "全局 数据发送重叠.vi" "数据接收超时指示灯"() -> (w359:bool)
                                n230 = Not(x=w359) -> (.not. x?=w360:bool)
                                }
                                frame "不判断" {
                                }
                                }
                                n231 = global read "全局 数据发送重叠.vi" "掉线指示灯"() -> (w352:bool)
                                n232 = global read "断电保存全局.vi" "数据重发"() -> (w346:bool)
                                n233 = Not(x=w352) -> (.not. x?=w351:bool)
                                n234 = Not(x=w346) -> (.not. x?=w347:bool)
                                n235 = Compound Arithmetic op=AND ("复合运算")(w347, w349, w351, w353) -> (w348:bool)
                                n236 = case shown="False" w348 {
                                tunnel: w355 -> [w363 w406]
                                tunnel: w354 -> [w365 w400]
                                tunnel: w356 -> [w367 w407]
                                tunnel: w346 -> [w366 _]
                                tunnel: w344 -> [w364 _]
                                frame False {
                                # "数据重发，或失败"
                                n237 = case shown="True" w366 {
                                tunnel: w367 -> [_ w371]
                                tunnel: w365 -> [_ w370]
                                tunnel: w364 -> [_ w369]
                                tunnel: w363 -> [_ w368]
                                frame False {
                                # "数据发送失败"
                                }
                                frame True {
                                # "数据重发"
                                n238 = case shown="True" w369 {
                                tunnel: w371 -> [w375 _]
                                tunnel: w370 -> [w373 w389]
                                tunnel: w368 -> [_ w390]
                                frame False {
                                # "重发完成恢复本地数据时间"
                                n239 = global read "全局1.vi" "配置文件队列名"() -> (w372:T2)
                                n240 = Unbundle By Name(w372) -> ("setini"=w382:string)
                                n241 = call <vilib>:"Application Directory.vi"() -> ("Application Directory"=w376:path)
                                n242 = Build Path(base path=w376, name or relative path=w382) -> (appended path=w377:path)
                                n243 = call <vilib>:"Open Config Data.vi"("configuration file path"=w377) -> ("error out"=w383:errorcluster, "refnum"=w378:T3)  [unwired: 8 in, 1 out]
                                n244 = global read "全局 水样时间.vi" "水样数据索引"() -> (w384:T4)
                                n245 = call-poly <vilib>:"Read Key.vi"("section"="线程一数据搜索起始时间", "error in (no error)"=w383, "key"=w375, "refnum"=w378) -> ("error out"=w381:errorcluster, "value"=w374:string, "refnum out"=w380:T3)  [unwired: 4 in, 1 out]
                                n246 = Cluster To Array(cluster=w384) -> (array=w385:string[])
                                n247 = call <vilib>:"Close Config Data.vi"("error in (no error)"=w381, "refnum"=w380) -> ()  [unwired: 8 in, 2 out]
                                n248 = Replace Array Subset(array=w385, new element=w374, index=w373) -> (w386:string[])
                                n249 = Array To Cluster(array=w386) -> (cluster=w387:T5)
                                n250 = global write "全局 水样时间.vi" "水样数据索引"(w387) -> ()
                                }
                                frame True {
                                # "数据拆分，继续重发"
                                n251 = call "日期时间字符串转换分钟数加一.vi"("data[0]"=w390) -> ("日期/时间字符串"=w388:string)  [unwired: 10 in]
                                n252 = global read "全局 水样时间.vi" "水样数据索引"() -> (w391:T4)
                                n253 = Cluster To Array(cluster=w391) -> (array=w392:string[])
                                n254 = Replace Array Subset(array=w392, new element=w388, index=w389) -> (w393:string[])
                                n255 = Array To Cluster(array=w393) -> (cluster=w394:T5)
                                n256 = global write "全局 水样时间.vi" "水样数据索引"(w394) -> ()
                                "数据拆分" <- TRUE
                                }
                                }
                                }
                                }
                                }
                                frame True {
                                # "保存本地"
                                n257 = global read "全局1.vi" "配置文件队列名"() -> (w396:T2)
                                n258 = call "日期时间字符串转换分钟数加一.vi"("枚举"=enum16{"分钟数加一", "秒数加一", "小时数加一"}."秒数加一", "data[0]"=w406) -> ("日期/时间字符串"=w399:string)  [unwired: 9 in]
                                n259 = Unbundle By Name(w396) -> ("setini"=w397:string)
                                n260 = global read "全局 水样时间.vi" "水样数据索引"() -> (w401:T4)
                                n261 = call <vilib>:"Application Directory.vi"() -> ("Application Directory"=w408:path)
                                n262 = Build Path(base path=w408, name or relative path=w397) -> (appended path=w409:path)
                                n263 = Cluster To Array(cluster=w401) -> (array=w402:string[])
                                n264 = call <vilib>:"Open Config Data.vi"("configuration file path"=w409) -> ("error out"=w411:errorcluster, "refnum"=w410:T3)  [unwired: 8 in, 1 out]
                                n265 = call "时间日期字符串至时间标识转换.vi"("时间日期字符串"=w399) -> ("时间标识"=→"数据发送起始时间":timestamp)  [unwired: 10 in]
                                n266 = call-poly <vilib>:"Write Key.vi"("section"="线程一数据搜索起始时间", "error in (no error)"=w411, "value"=w399, "key"=w407, "refnum"=w410) -> ("error out"=w413:errorcluster, "refnum out"=w412:T3)  [unwired: 4 in, 1 out]
                                n267 = Replace Array Subset(array=w402, new element=w399, index=w400) -> (w403:string[])
                                n268 = Array To Cluster(array=w403) -> (cluster=w404:T5)
                                n269 = call <vilib>:"Close Config Data.vi"("error in (no error)"=w413, "refnum"=w412) -> ()  [unwired: 8 in, 2 out]
                                n270 = global write "全局 水样时间.vi" "水样数据索引"(w404) -> ()
                                }
                                }
                              }
                            }
                          }
                        }
                      }
                    }
                  }
                }
              }
            }
            frame #1 {
            }
          }
        }
        frame True {
          # "数据整点触发，整条发送"
          n271 = flat-sequence {
            frame #0 {
              n272 = global read "断电保存全局.vi" "数据发送通道"() -> (w416:enum16{"TCP", "VISA"})
              n273 = global read "断电保存全局.vi" "MN"() -> (w418:string)
              n274 = global read "断电保存全局.vi" "PW"() -> (w417:string)
              n275 = call "数据全参数一起发送整点触发.vi"("数据发送通道"=w416, "PW"=w417, "MN"=w418) -> ()  [unwired: 8 in]
            }
            frame #1 {
              w419 = FALSE ("主动上报数据中")
              n276 = global write "全局 数据发送重叠.vi" "主动上报数据中"(w419) -> ()
              n277 = global write "全局1.vi" "实时小时数据上传"(w419) -> ()
            }
          }
        }
      }
    }
  }
  "error out" <- w3
